vi "Test DI Change Detection.vi"() -> ()   [LabVIEW 2015]
uses:
  <vilib>/DAQmx/create/channels.llb/DAQmx Create Channel (DI-Digital Input).vi
  <vilib>/DAQmx/configure/timing.llb/DAQmx Timing (Change Detection).vi
panel:
  in  "lines":tag="PXI1Slot2/port0/line0"
  in  "stop":bool
  out "Numeric 2":i32
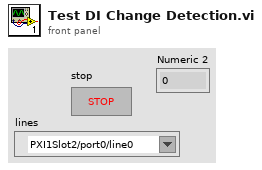
[diagram p1: front panel]
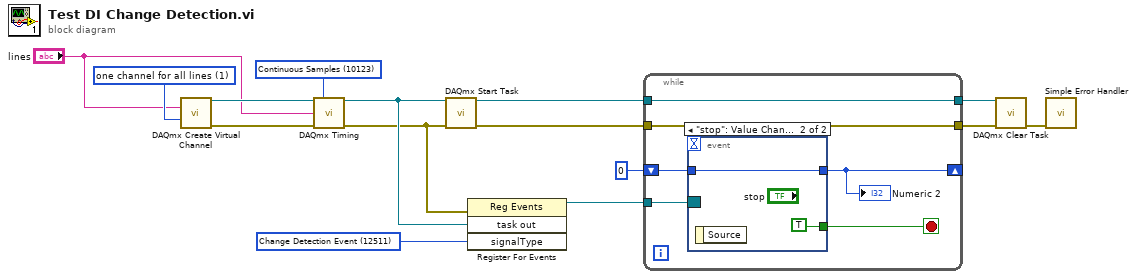
[diagram p0: block diagram]
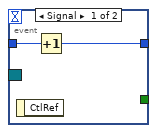
[diagram p2: hidden frame]
diagram:
  w9 = 12511 items=["Sample Complete Event"=12530, "Counter Output Event"=12494, "Change Detection Event"=12511, "Sample Clock"=12487] ("signalType")
  w12 = 10123 items=["Finite Samples"=10178, "Continuous Samples"=10123, "Hardware Timed Single Point"=12522] ("sample mode")
  w15 = 1 items=["one channel for each line", "one channel for all lines"] ("line grouping")
  n1 = call-poly <vilib>:"DAQmx Create Virtual Channel.vi"("lines"="lines", "line grouping"=w15) -> ("task out"=w7:refnum<k21>, "error out"=w14:errorcluster)  [unwired: 12 in]
  n2 = call-poly <vilib>:"DAQmx Timing.vi"("task/channels in"=w7, "sample mode"=w12, "rising edge physical channels"="lines", "error in"=w14) -> ("task out"=w10:refnum<k21>, "error out"=w5:errorcluster)  [unwired: 10 in]
  n3 = call <vilib>:"DAQmx Start Task.vi"("task/channels in"=w10, "error in"=w5) -> ("task out"=w11:refnum<k21>, "error out"=w6:errorcluster)  [unwired: 12 in]
  n4 = register-events(error in=w5, w10, w9) -> (reference out=w8:refnum<event-registration>)  [unwired: 1 in, 1 out]
  n5 = while {
    tunnel: w11 -> [w18]
    tunnel: w6 -> [w17]
    tunnel: w8 -> [w21]
    shift-right: [w19] -> _
    shift-left: 0 -> [w20]
    tunnel: [w18] -> w3
    tunnel: [w17] -> w2
    stop <- w16 stop-if-true
    n6 = event shown="[1] \"stop\": Value Change" {
      selector: w21 -> [_ _]
      dyn-events: _ -> [_ _]
      timeout: _ -> [_ _]
      tunnel: w20 -> [w23 w24]
      tunnel: [w22 w24] -> w19
      tunnel: [_ TRUE] -> w16
      event Signal {
        n7 = event-data() -> ()  [unwired: 1 in, 1 out]
        n8 = Increment(x=w23) -> (x+1=w22:i32)
      }
      event "stop": Value Change {
        n9 = event-data() -> ()  [unwired: 1 in, 1 out]
      }
    }
    "Numeric 2" <- w19
  }
  n10 = call <vilib>:"DAQmx Clear Task.vi"("task in"=w3, "error in"=w2) -> ("error out"=w13:errorcluster)  [unwired: 13 in]
  n11 = call <vilib>:"Simple Error Handler.vi"("error in (no error)"=w13) -> ()  [unwired: 4 in, 5 out]
